vi "New.vi"(11 "File Path":path) -> (3 "FileConfig.lvclass":refnum<class "FileConfig.lvclass">)   [LabVIEW 2019, in "FileConfig.lvclass"]
uses:
  FileConfig.lvclass
  FileConfig.lvclass/FileConfig.ctl
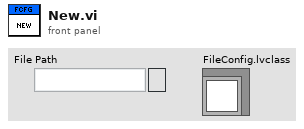
[diagram p1: front panel]
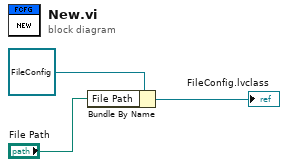
[diagram p0: block diagram]
diagram:
  n1 = Bundle By Name(cluster=refnum<class "FileConfig.lvclass"> refnum ("FileConfig.lvclass"), "File Path"="File Path") -> (→"FileConfig.lvclass":refnum<class "FileConfig.lvclass">)
